vi "Select Mask.vi"(5 "Read \nImage":T2(plugin-control)=refnum, 6 "Prompt":string="Select Left Mask", 7 "error in":errorcluster) -> (0 "mask":T2(plugin-control), 1 "Masked \nImage":T2(plugin-control), 2 "Annulus":T1={"Center X"=982, "Center Y"=650, "Inner Radius"=309, "Outer Radius"=405, "Start Angle"=90.0, "End Angle"=180.0} {"End Angle" format="%.2f"; "Start Angle" format="%.2f"; "Center X" scale=0.0..1024.0}, 3 "error out":errorcluster, 4 "Cancelled":bool)   [LabVIEW 2013, in "Image Processing.lvlib"]
uses:
  Image Processing.lvlib
  <vilib>/vision/NI_Vision_Development_Module.lvlib
panel:
  in  "Annulus Angles":cluster{"Start Angle":dbl, "End Angle":dbl}={"Start Angle"=0.0, "End Angle"=90.0}
  in  "Set Window Coordinates":cluster{"X Position":i32, "Y Position":i32}={"X Position"=0, "Y Position"=100}
  out "Window Coordinates":cluster{"X Position":i32, "Y Position":i32}={"X Position"=0, "Y Position"=100}
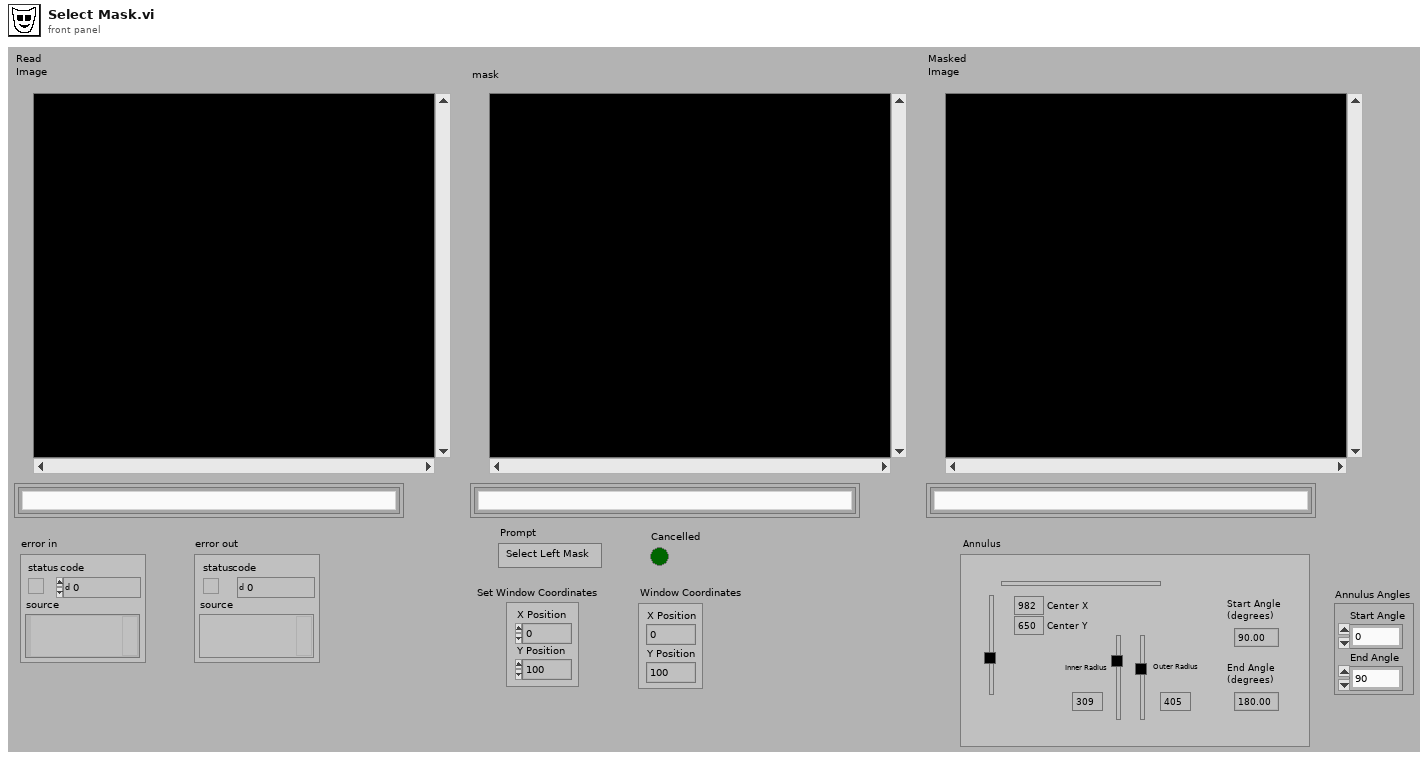
[diagram p1: front panel]
types:
  T1 = typedef "IMAQ Circle" = cluster{"Center X":i32, "Center Y":i32, "Inner Radius":i32, "Outer Radius":i32, "Start Angle":dbl, "End Angle":dbl}
  T2 = typedef "IMAQ Image.ctl" = refnum<image>
  T3 = typedef "ROI Descriptor" = cluster{"Global Rectangle":i32[], "Contours":cluster{"ID":enum32{"External", "Internal"}, "Type":u32, "Coordinates":i32[]}[]}
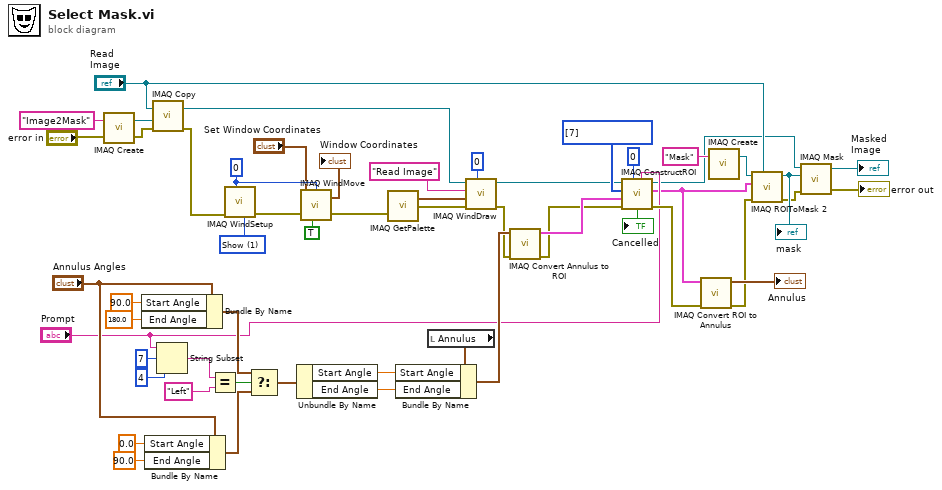
[diagram p0: block diagram]
diagram:
  w10 = u32[] [7] items=["No Selection", "Point", "Line", "Rectangle", "Oval", "Polygon", "Freehand Region", "Annulus", "Zoom", "Pan", "Broken Line", "Freehand Line", "Rotated Rectangle"] ("Tools")
  w45 = 1 items=["Hide", "Show", "No change"] ("Scrollbars (No change)")
  w41 = 0 ("Window Number (0...15)")
  n1 = call "IMAQ Create"("Image Name"="Image2Mask", "error in (no error)"="error in") -> ("New Image"=w37:T2, "error out"=w33:errorcluster)  [unwired: 3 in]
  n2 = Bundle By Name(cluster="Annulus Angles", "Start Angle"=90.0, "End Angle"=180.0) -> (w21:cluster{"Start Angle":dbl, "End Angle":dbl})
  n3 = Bundle By Name(cluster="Annulus Angles", "Start Angle"=0.0, "End Angle"=90.0) -> (w17:cluster{"Start Angle":dbl, "End Angle":dbl})
  n4 = call "IMAQ Copy"("error in (no error)"=w33, "Image Dst"=w37, "Image Src"="Read \nImage") -> ("error out"=w31:errorcluster, "Image Dst Out"=w35:T2)  [unwired: 3 in]
  n5 = String Subset(string="Prompt", offset (0)=7, length (rest)=4 ("length (rest)")) -> (substring=w25:string)
  n6 = Equal?(x=w25, y="Left") -> (x = y?=w24:bool)
  n7 = call "IMAQ WindSetup"("Scrollbars (No change)"=w45, "Window Number (0...15)"=w41, "error in (no error)"=w31) -> ("error out"=w43:errorcluster)  [unwired: 8 in]
  n8 = Select(t=w21, s=w24, f=w17) -> (s? t:f=w16:cluster{"Start Angle":dbl, "End Angle":dbl})
  n9 = Unbundle By Name(w16) -> ("Start Angle"=w15:dbl, "End Angle"=w14:dbl)
  n10 = call "IMAQ WindMove"("Window Number (0...15)"=w41, "Coordinates (screen)"="Set Window Coordinates", "Get/Set Status? (Set)"=TRUE, "error in (no error)"=w43) -> ("Coordinates (screen)"=→"Window Coordinates":cluster{"X Position":i32, "Y Position":i32}, "error out"=w40:errorcluster)  [unwired: 1 in]
  n11 = call "IMAQ GetPalette"("error in (no error)"=w40) -> ("Color Palette"=w47:cluster{"Red":u8, "Green":u8, "Blue":u8}[], "error out"=w46:errorcluster)  [unwired: 4 in]
  n12 = local read "Annulus"() -> (w30:T1)
  n13 = Bundle By Name(cluster=w30, "Start Angle"=w15, "End Angle"=w14) -> (w29:T1)
  n14 = call "IMAQ WindDraw"("Window Number (0...15)"=0, "error in (no error)"=w46, "Color Palette"=w47, "Title"="Read Image", "Image"=w35) -> ("error out"=w13:errorcluster, "Image Out (duplicate)"=w7:T2)  [unwired: 1 in, 4 out]
  n15 = call "IMAQ Convert Annulus to ROI"("error in (no error)"=w13, "Annulus"=w29) -> ("error out"=w8:errorcluster, "ROI Descriptor"=w9:T3)  [unwired: 7 in]
  n16 = call "IMAQ ConstructROI"("Prompt"="Prompt", "Window Number (-1...15)"=0 ("Window Number (0...15)"), "error in (no error)"=w8, "ROI Descriptor In (None)"=w9, "Tools"=w10, "Image"=w7) -> ("error out"=w12:errorcluster, "Cancel"=→"Cancelled":bool, "ROI Descriptor Out"=w2:T3, "Image Out (duplicate)"=w5:T2)  [unwired: 2 in]
  n17 = call "IMAQ Convert ROI to Annulus"("error in (no error)"=w12, "ROI Descriptor"=w2) -> ("error out"=w1:errorcluster, "Annulus"=→"Annulus":T1)  [unwired: 7 in]
  n18 = call "IMAQ Create"("Image Name"="Mask") -> ("New Image"=w50:T2)  [unwired: 3 in, 2 out]
  n19 = call "IMAQ ROIToMask 2"("Image Model"="Read \nImage", "error in (no error)"=w1, "ROI Descriptor"=w2, "Image"=w50) -> ("error out"=w49:errorcluster, "Image Out"=w53:T2)  [unwired: 5 in, 1 out]
  "mask" <- w53
  n20 = call "IMAQ Mask"("error in (no error)"=w49, "Image Mask"=w53, "Image Src"=w5) -> ("error out"=→"error out":errorcluster, "Image Dst Out"=→"Masked \nImage":T2)  [unwired: 1 in, 1 out]
